vi "Client ATM machine.vi"() -> ()   [LabVIEW 2020]
uses:
  Sub VIs/Enum (Client).ctl
  <vilib>/regexp/Match Regular Expression.xnode
panel:
  out "Account no":string
  out "error out":errorcluster
  out "Data from server side":string caption="data out"
  out "First Name":string
  out "Balance":dbl
  out "Last Name":string
  in  "Client ATM Machine UI":enum32{"Page 1"}(tab)
  in  "User Input":string
  in  "Card Simulator":bool
  in  "Enter":bool
  out "ATM Message":string
  out "Left Menu":T1
  out "Right Menu":T2
  in  "Right Button":T3
  in  "Left Button":T4
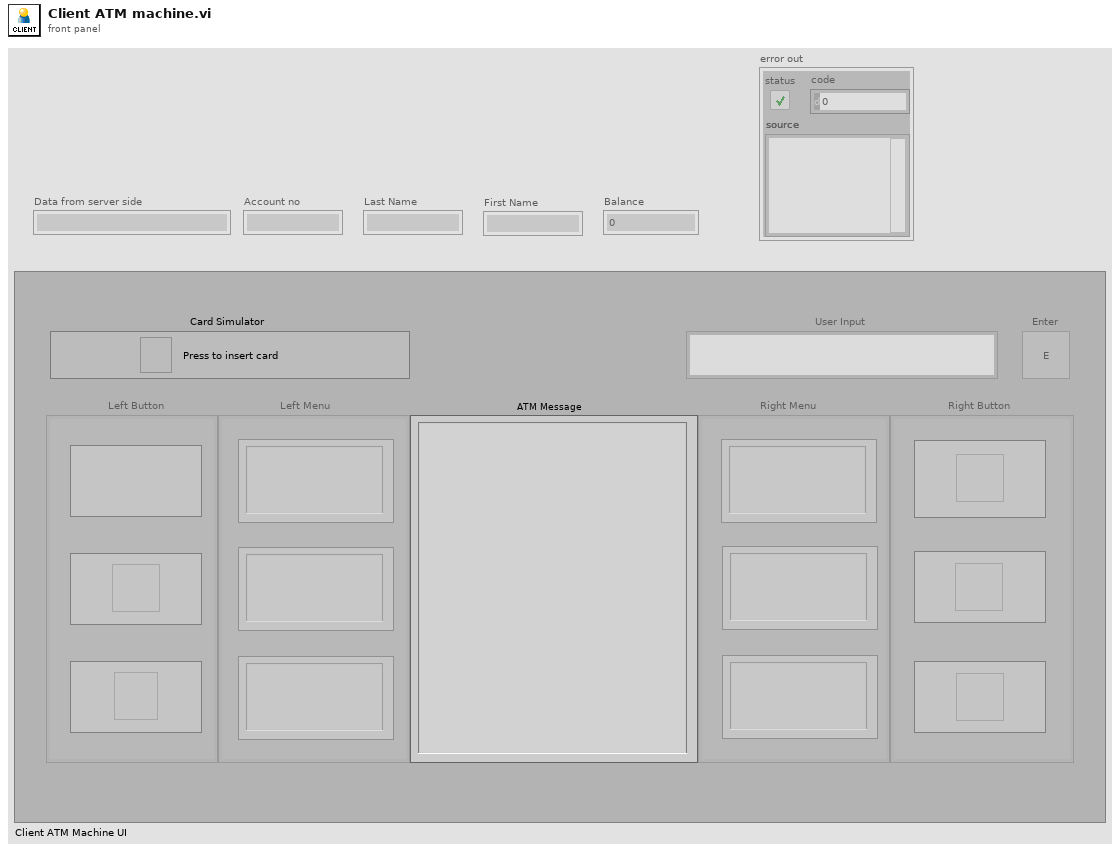
[diagram p1: front panel]
types:
  T1 = cluster{"Left Menu 3":string, "Left Menu 2":string, "Left Menu 4":string}
  T2 = cluster{"Right Menu 2":string, "Right Menu":string, "Right Menu 3":string}
  T3 = cluster{"Deposit":bool, "Withdraw":bool, "Fast Cash":bool}
  T4 = cluster{"None":bool, "Bank Inquires":bool, "Return Card and Terminate ":bool}
  T5 = typedef "Enum (Client).ctl" = enum16{"Start", "Idle", "Actions", "Empty Check", "Data Transmission", "Update File"}
  T6 = enum8{"Enabled", "Disabled", "Disabled and Grayed Out"}
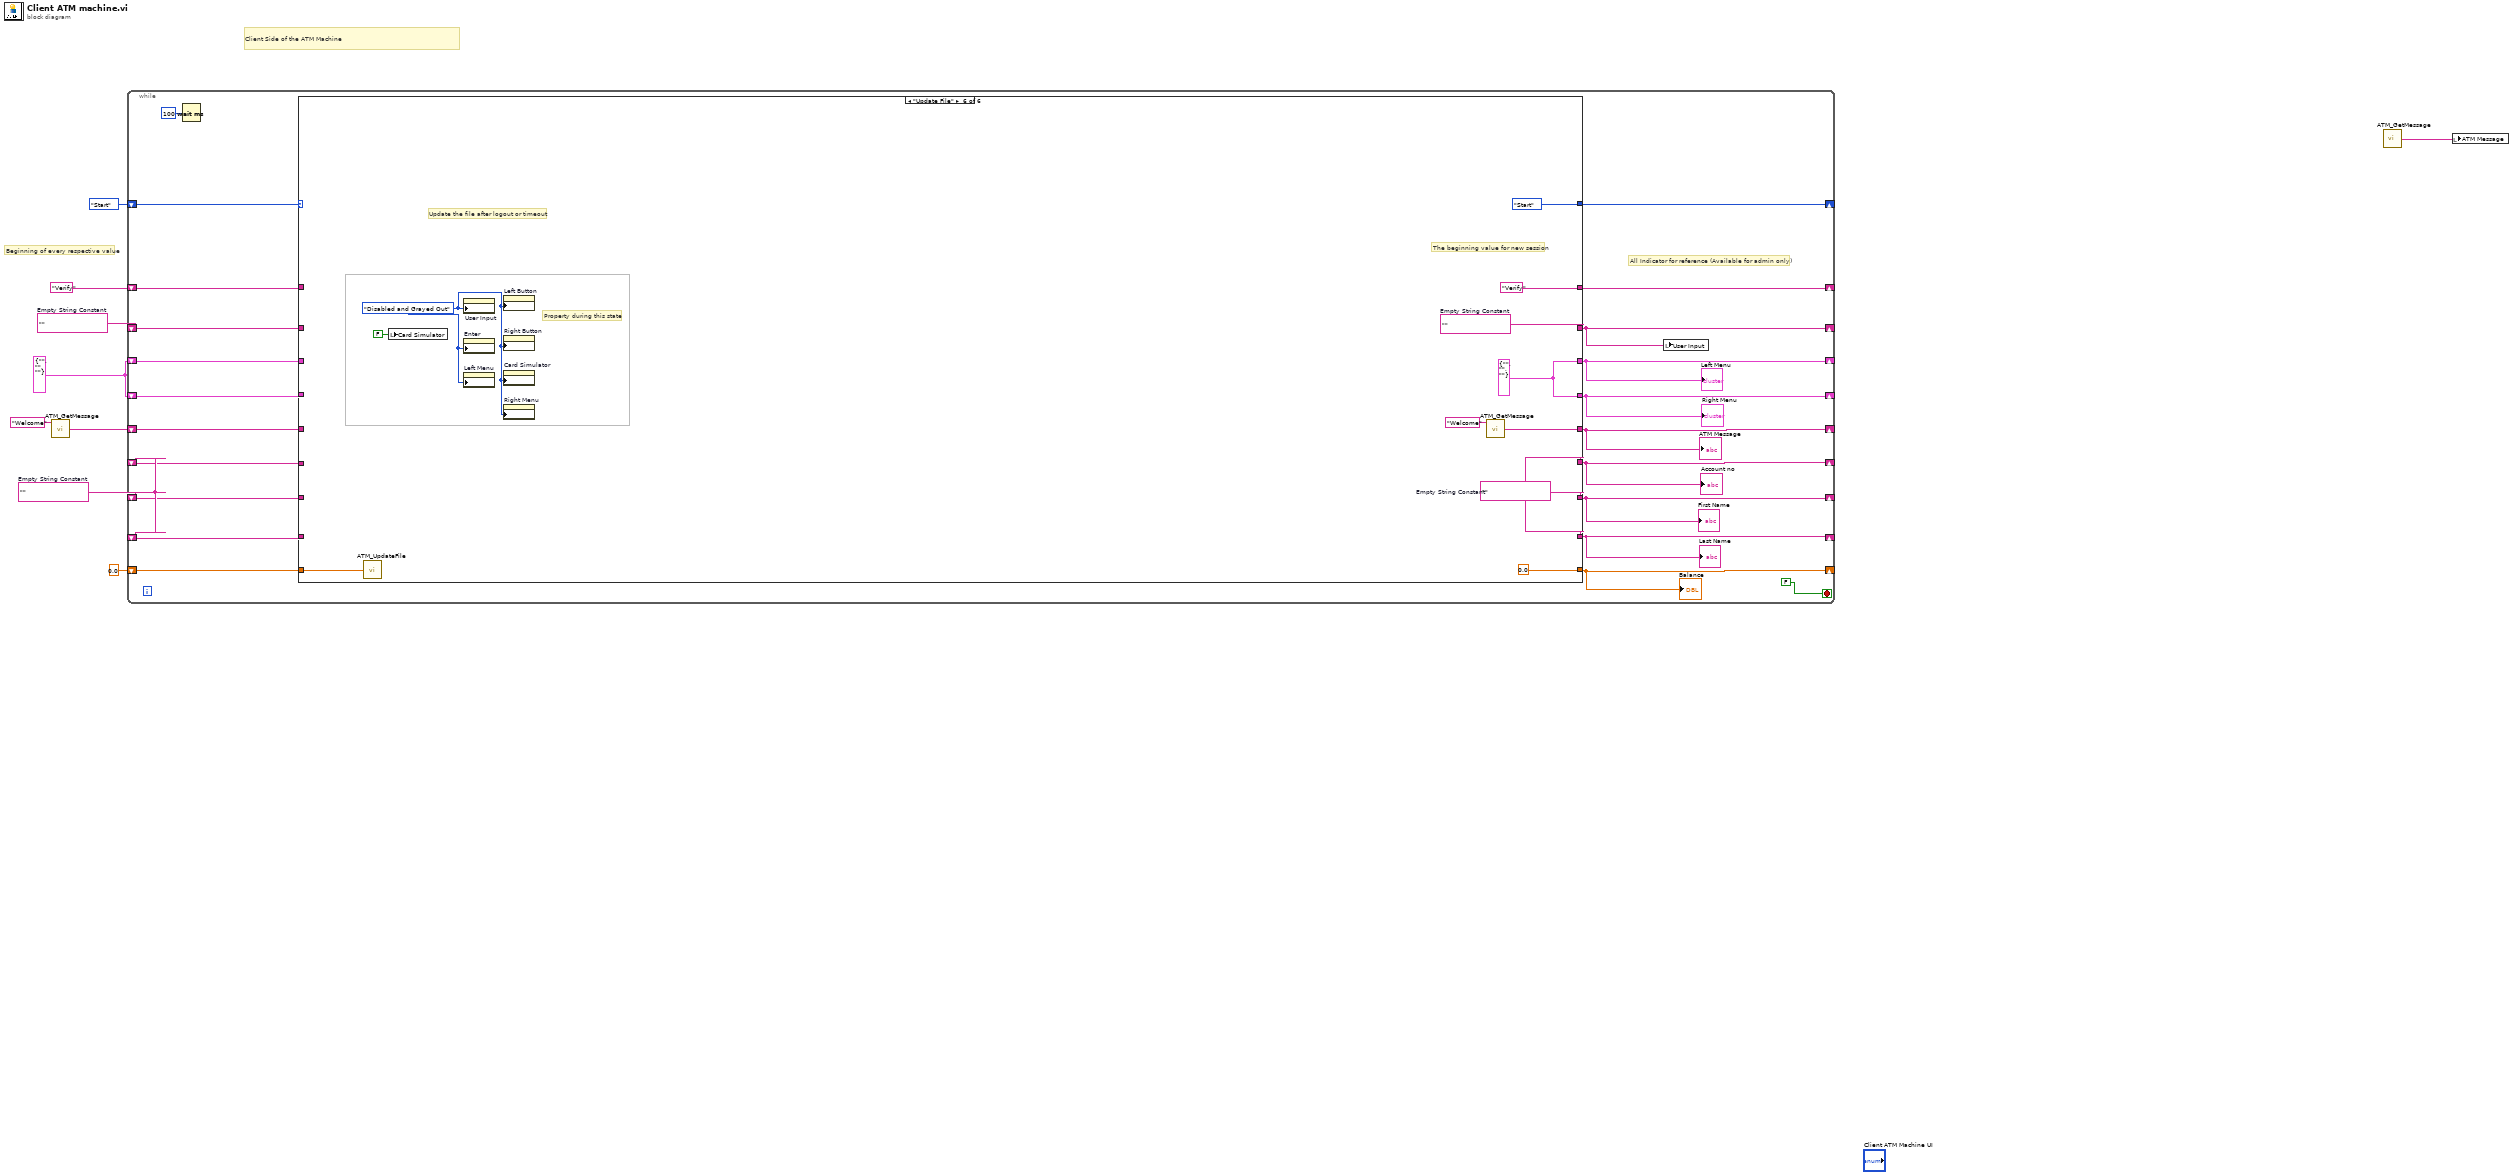
[diagram p0: block diagram]
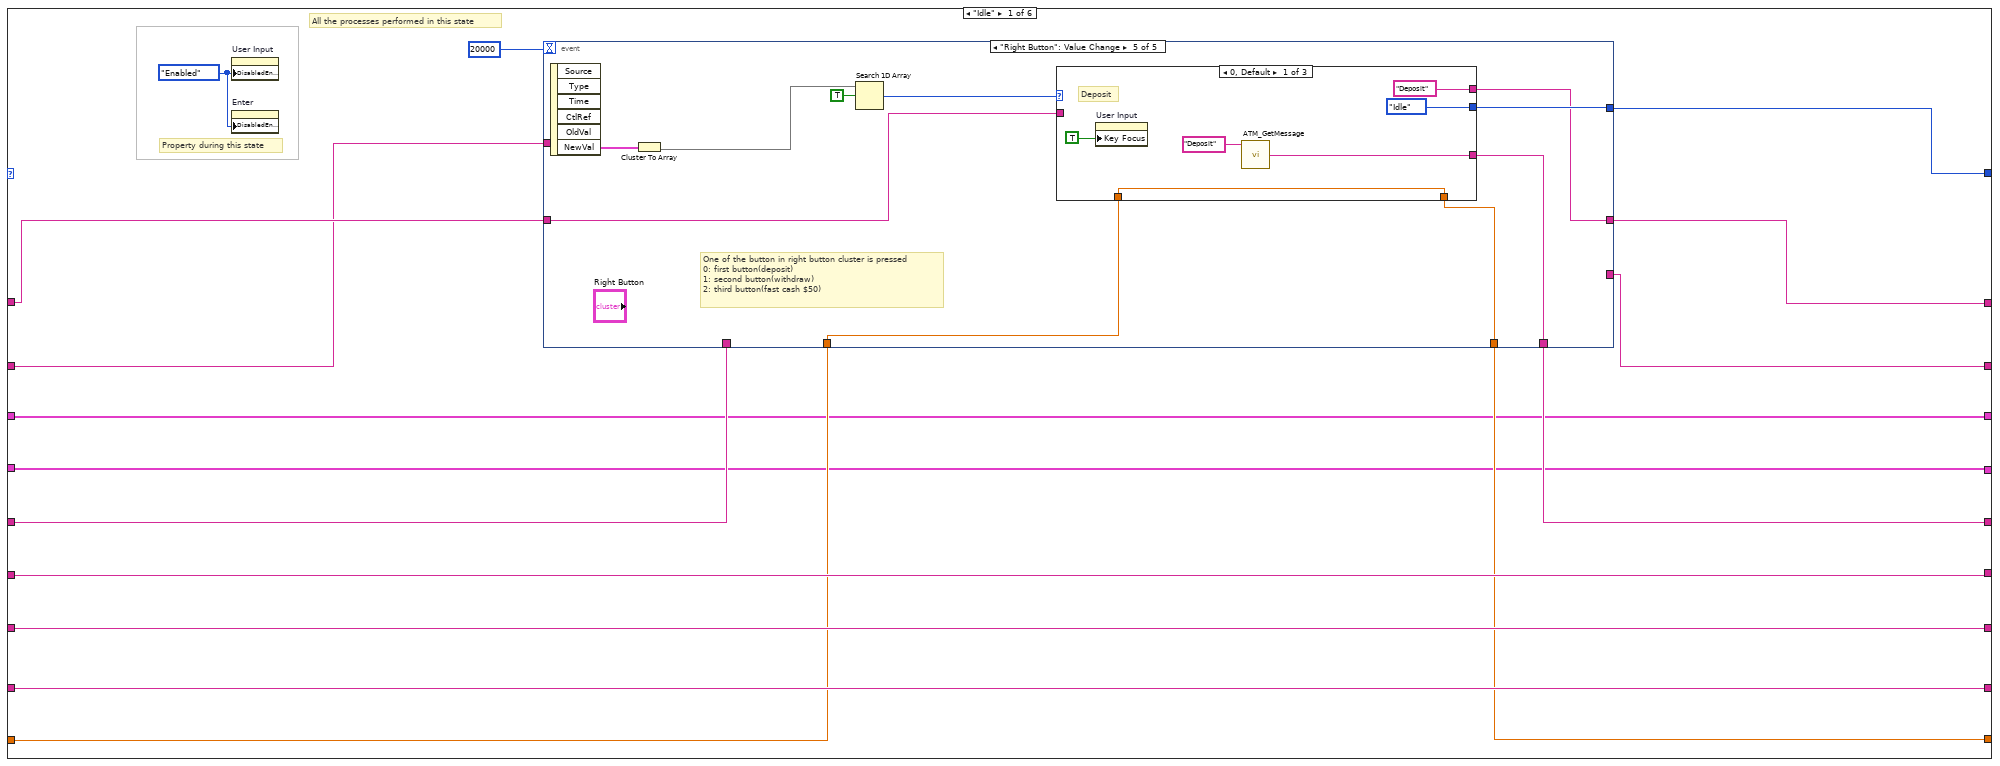
[diagram p2: hidden frame]
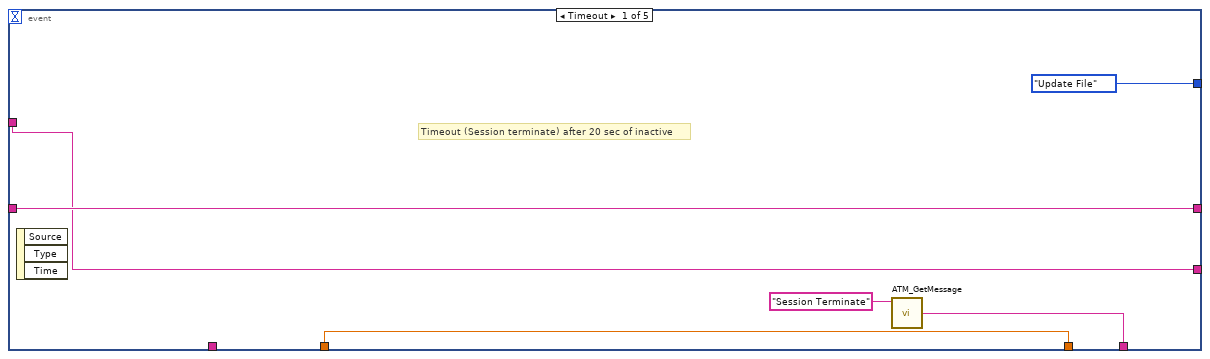
[diagram p3: hidden frame]
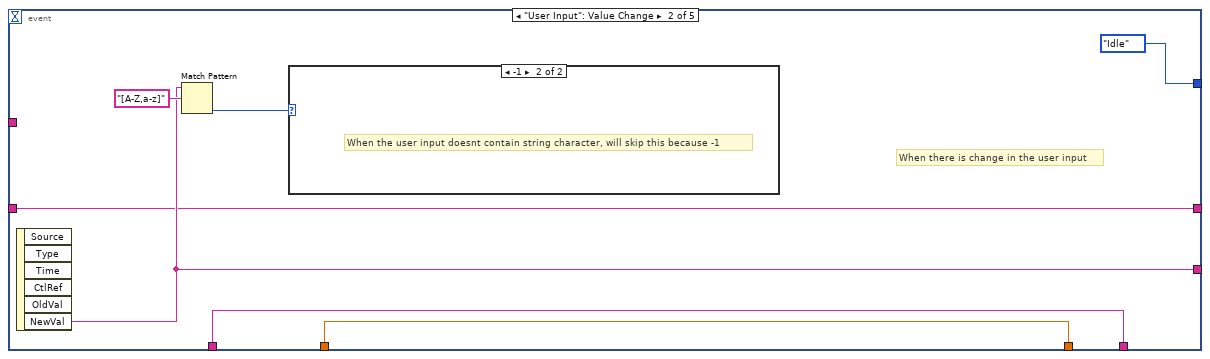
[diagram p4: hidden frame]
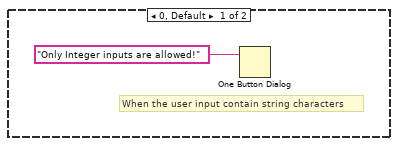
[diagram p5: hidden frame]
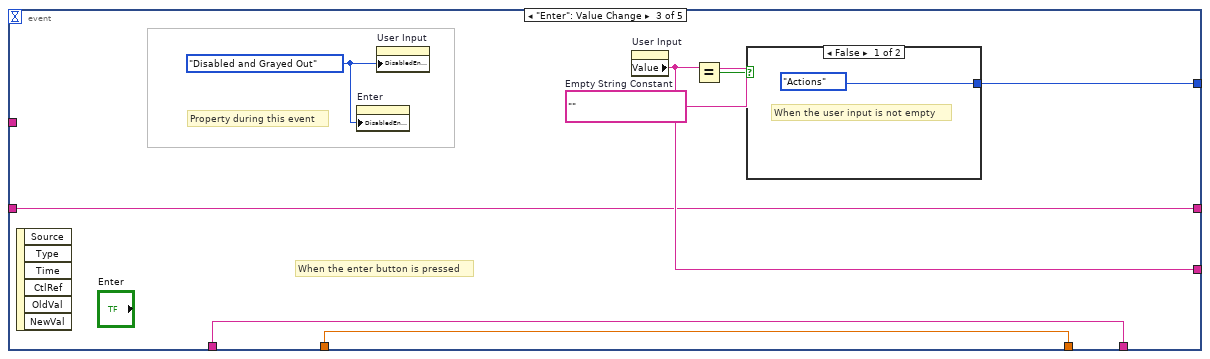
[diagram p6: hidden frame]
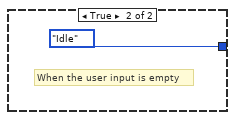
[diagram p7: hidden frame]
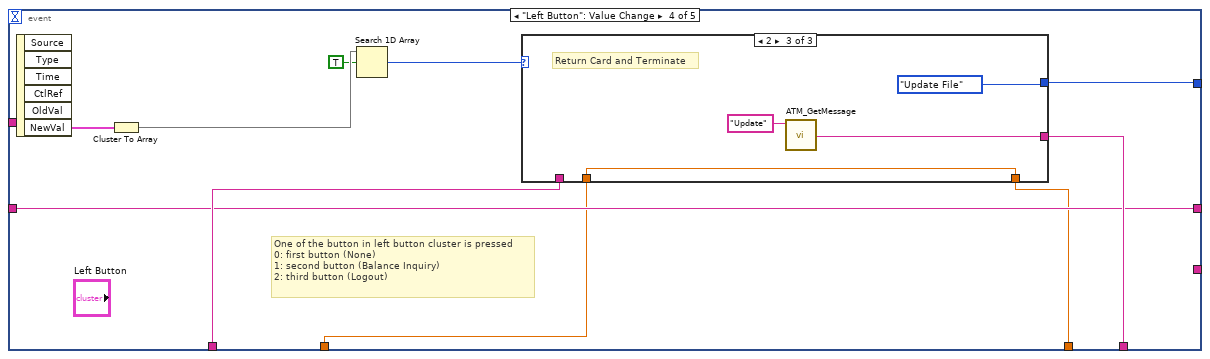
[diagram p8: hidden frame]
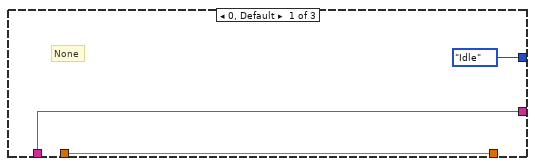
[diagram p9: hidden frame]
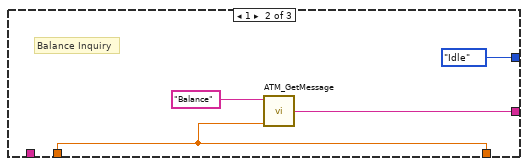
[diagram p10: hidden frame]
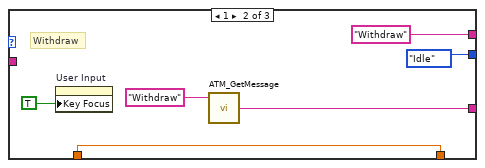
[diagram p11: hidden frame]
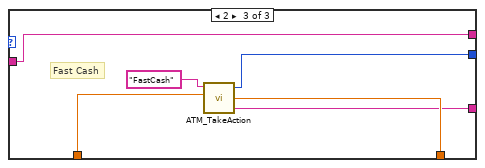
[diagram p12: hidden frame]
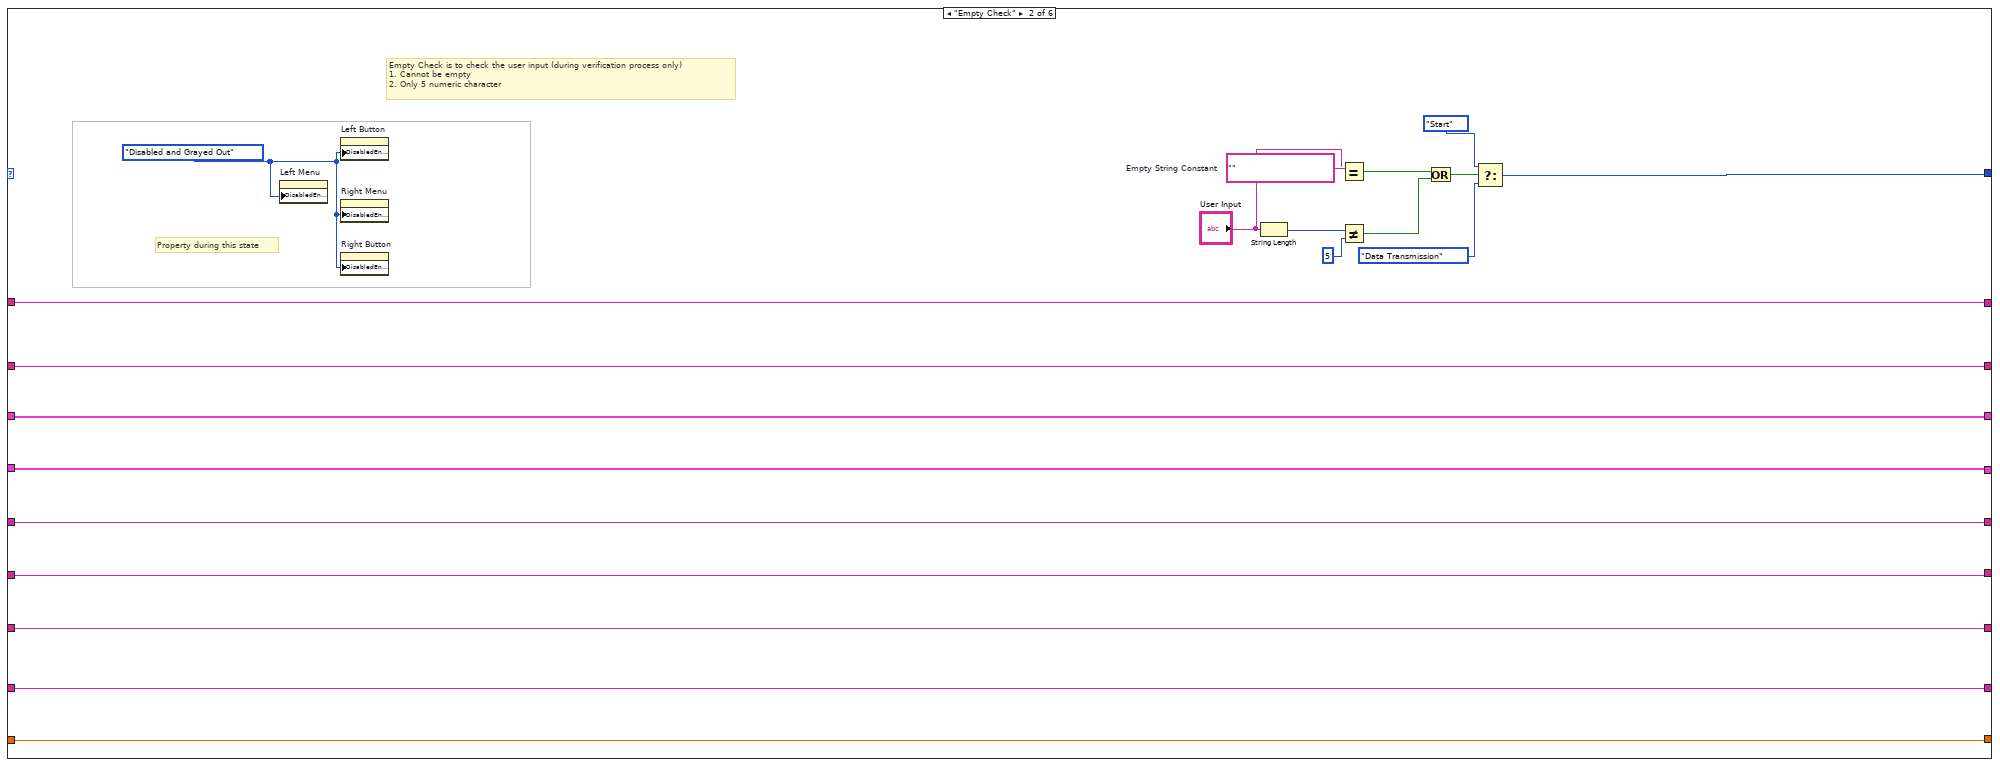
[diagram p13: hidden frame]
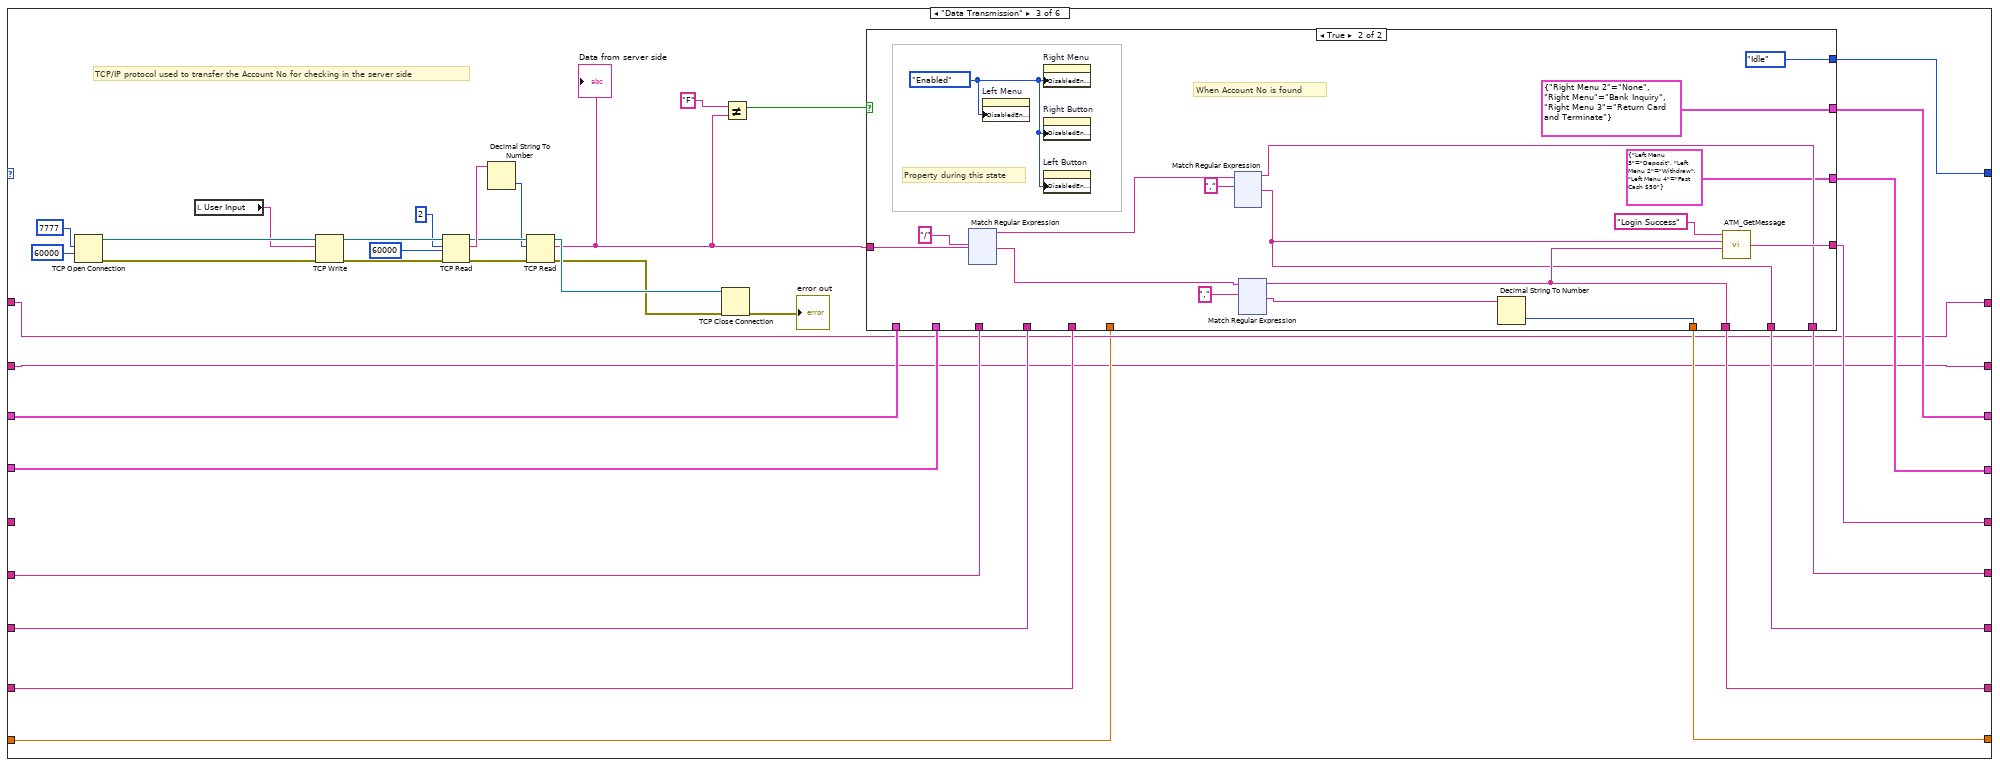
[diagram p14: hidden frame]
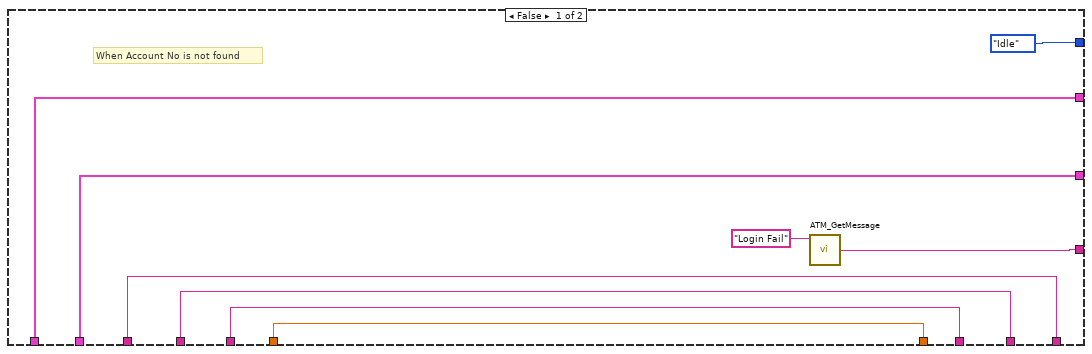
[diagram p15: hidden frame]
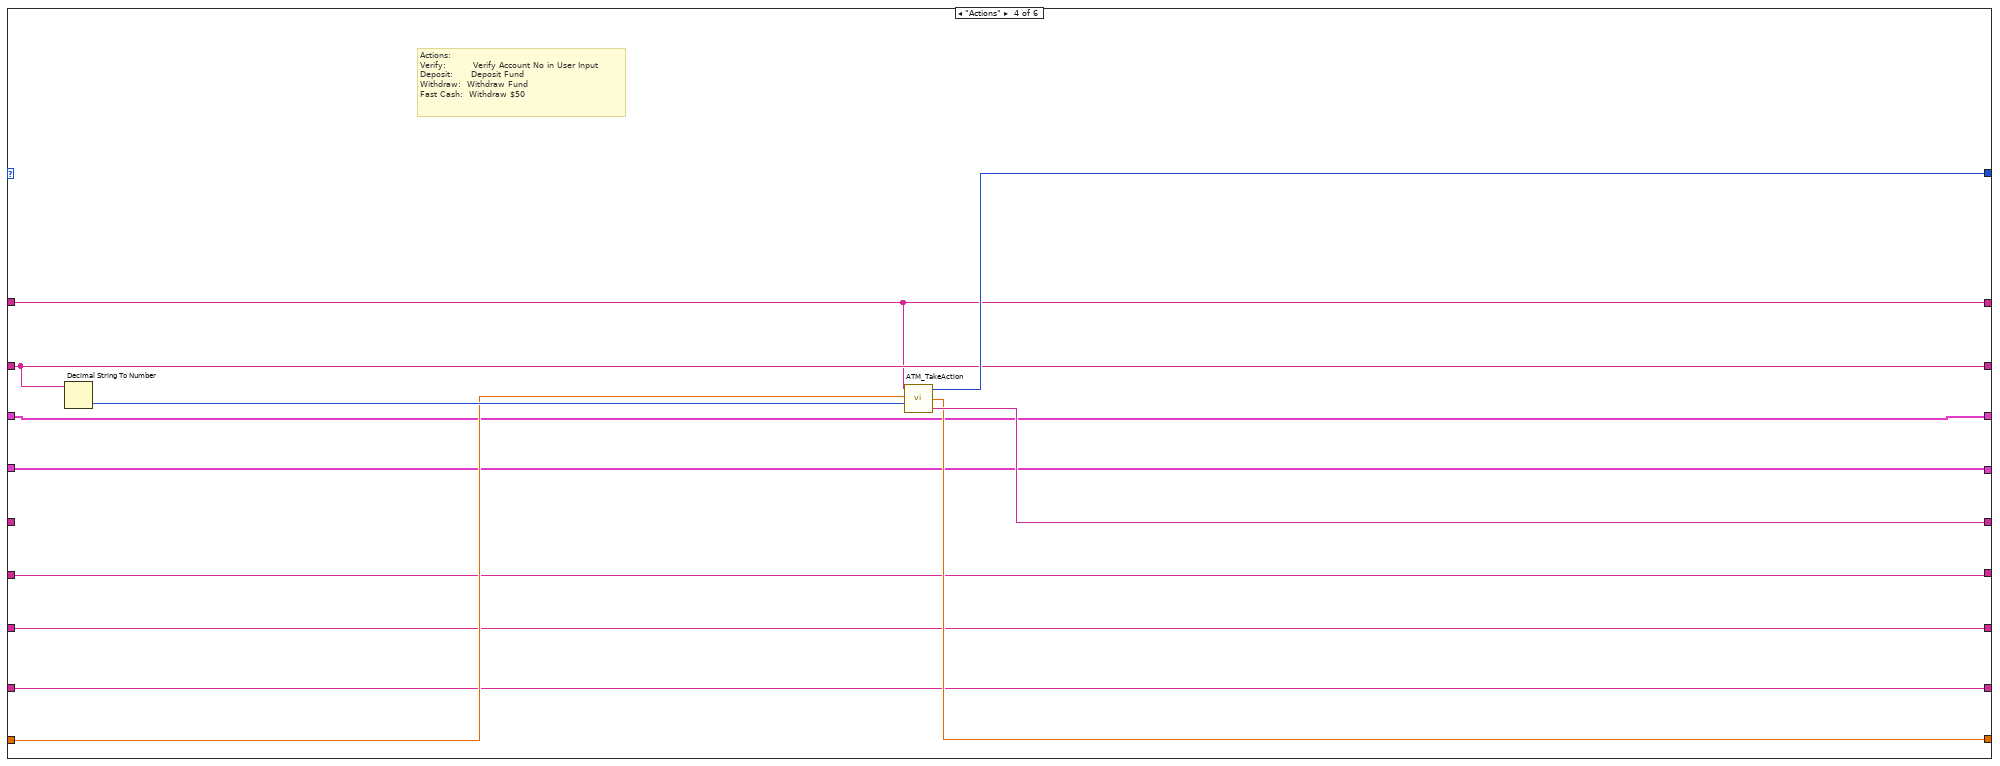
[diagram p16: hidden frame]
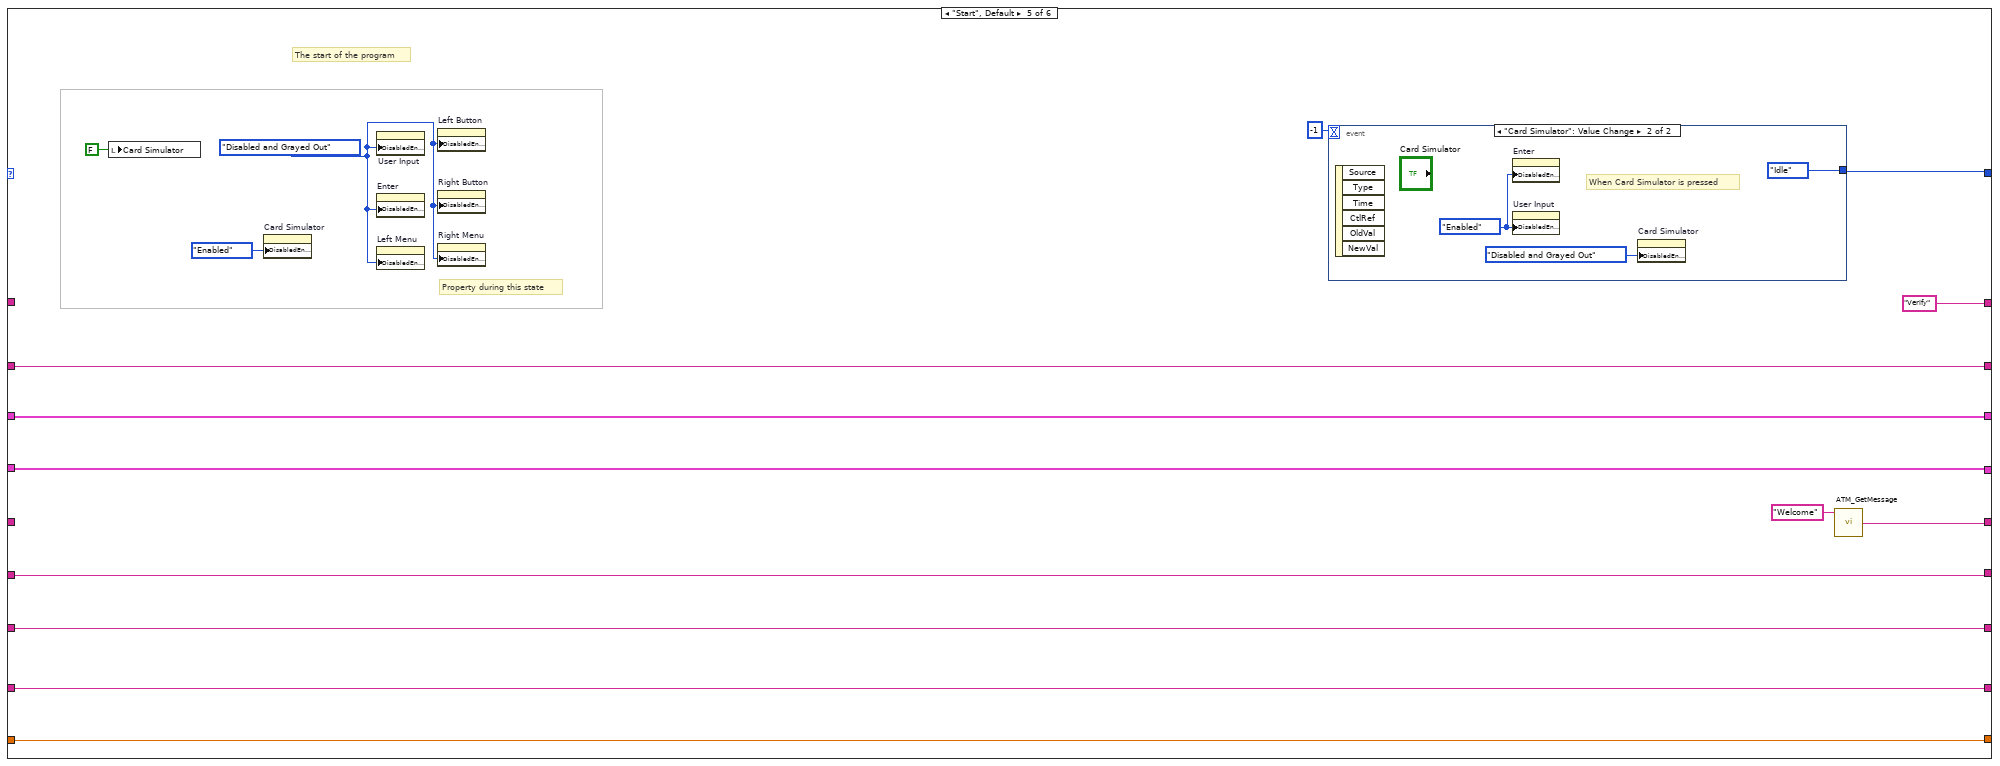
[diagram p17: hidden frame]
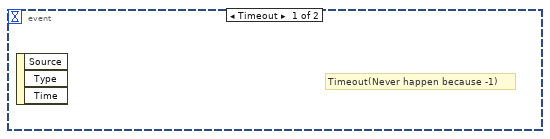
[diagram p18: hidden frame]
diagram:
  w1 = ""  # Empty String Constant
  w2 = ""  # Empty String Constant
  w6 = T2 {"Right Menu 2"="", "Right Menu"="", "Right Menu 3"=""} ("Right Menu")
  # "Client Side of the ATM Machine"
  # "Beginning of every respective value"
  n1 = call "ATM_GetMessage.vi"("Message Type"="Welcome") -> ("ATM Message"=w4:string)  [unwired: 4 in]
  n2 = while {
    shift-right: [w19] -> _
    shift-left: Enum_(Client)."Start" -> [w27]
    shift-right: [w28] -> _
    shift-left: "Verify" -> [w29]
    shift-right: [w16] -> _
    shift-left: w6 -> [w25]
    shift-right: [w18] -> _
    shift-left: w6 -> [w26]
    shift-right: [w20] -> _
    shift-left: 0.0 ("Balance") -> [w21]
    shift-right: [w13] -> _
    shift-left: w2 -> [w22]
    shift-right: [w15] -> _
    shift-left: w2 -> [w23]
    shift-right: [w17] -> _
    shift-left: w4 -> [w24]
    shift-right: [w11] -> _
    shift-left: w2 -> [w14]
    shift-right: [w10] -> _
    shift-left: w1 -> [w12]
    stop <- FALSE stop-if-true
    # "All Indicator for reference (Available for admin only)"
    n3 = Wait (ms)(milliseconds to wait=u32 100) -> ()  [unwired: 1 out]
    n4 = case shown="\"Update File\"" w27 {
      tunnel: [w47 w132 w141 w552 w560 Enum_(Client)."Start"] -> w19
      tunnel: w29 -> [w39 w131 w147 w544 _ _]
      tunnel: [w34 w131 w147 w544 "Verify" "Verify"] -> w28
      tunnel: [w44 w126 w159 w546 w564 w579] -> w13
      tunnel: [w46 w125 w158 w547 w563 w579] -> w15
      tunnel: [w43 w124 w157 w548 w567 w579] -> w11
      tunnel: [w42 w123 w156 w551 w568 0.0 ("Balance")] -> w20
      tunnel: [w36 w129 w155 w549 w566 w581] -> w18
      tunnel: [w37 w128 w154 w550 w565 w581] -> w16
      tunnel: w26 -> [w36 w129 w152 w549 w566 _]
      tunnel: w25 -> [w37 w128 w151 w550 w565 _]
      tunnel: w24 -> [w38 w127 _ _ _ _]
      tunnel: [w40 w127 w153 w553 w556 w574] -> w17
      tunnel: w23 -> [w46 w125 w149 w547 w563 _]
      tunnel: w22 -> [w44 w126 w150 w546 w564 _]
      tunnel: w21 -> [w41 w123 w146 w554 w568 w584]
      tunnel: w14 -> [w43 w124 w148 w548 w567 _]
      tunnel: w12 -> [w32 w122 w145 w545 w562 _]
      tunnel: [w35 w122 w145 w545 w562 w578] -> w10
      frame "Idle" {
        w33 = T6."Enabled" ("Disabled")
        # "Property during this state"
        # "All the processes performed in this state"
        n5 = property on="User Input" class="Str"("DisabledEnum"=w33) -> ()  [unwired: 2 in, 2 out]
        n6 = property on="Enter" class="Bool"("DisabledEnum"=w33) -> ()  [unwired: 2 in, 2 out]
        n7 = event shown="[4] \"Right Button\": Value Change" {
          selector: _ -> [_ _ _ _ _]
          dyn-events: _ -> [_ _ _ _ _]
          timeout: 20000 -> [_ _ _ _ _]
          tunnel: [Enum_(Client)."Update File" Enum_(Client)."Idle" w66 w77 w98] -> w47
          tunnel: w41 -> [w49 w58 w68 w73 w97]
          tunnel: [w49 w58 w68 w72 w96] -> w42
          tunnel: [w51 w57 w69 w76 w95] -> w40
          tunnel: w39 -> [w50 w55 w62 w74 w94]
          tunnel: w38 -> [_ w57 w69 w75 _]
          tunnel: [w48 w56 w64 _ _] -> w35
          tunnel: [w50 w55 w62 w74 w93] -> w34
          tunnel: w32 -> [w48 _ _ _ _]
          event Timeout {
            # "Timeout (Session terminate) after 20 sec of inactive"
            n8 = event-data() -> ()  [unwired: 1 in, 3 out]
            n9 = call "ATM_GetMessage.vi"("Message Type"="Session Terminate") -> ("ATM Message"=w51:string)  [unwired: 4 in]
          }
          event "User Input": Value Change {
            # "When there is change in the user input"
            n10 = event-data() -> ("NewVal"=w56:string)  [unwired: 1 in, 5 out]
            n11 = Match Pattern(string=w56, regular expression="[A-Z,a-z]") -> (offset past match=w60:i32)  [unwired: 1 in, 3 out]
            n12 = case shown="-1" w60 {
              frame 0, Default {
                # "When the user input contain string characters"
                n13 = One Button Dialog(message="Only Integer inputs are allowed!") -> ()  [unwired: 1 in, 1 out]
              }
              frame -1 {
                # "When the user input doesnt contain string character, will skip this because -1"
              }
            }
          }
          event "Enter": Value Change {
            w63 = T6."Disabled and Grayed Out" ("Disabled")
            w67 = ""  # Empty String Constant
            # "Property during this event"
            # "When the enter button is pressed"
            n14 = event-data() -> ()  [unwired: 1 in, 6 out]
            n15 = property on="Enter" class="Bool"("DisabledEnum"=w63) -> ()  [unwired: 2 in, 2 out]
            n16 = property on="User Input" class="Str"("DisabledEnum"=w63) -> ()  [unwired: 2 in, 2 out]
            n17 = property on="User Input" class="Str"() -> ("Value"=w64:string)  [unwired: 2 in, 2 out]
            n18 = Equal?(x=w64, y=w67) -> (x = y?=w65:bool)
            n19 = case shown="False" w65 {
              tunnel: [Enum_(Client)."Actions" Enum_(Client)."Idle"] -> w66
              frame False {
                # "When the user input is not empty"
              }
              frame True {
                # "When the user input is empty"
              }
            }
          }
          event "Left Button": Value Change {
            # "One of the button in left button cluster is pressed\n0: first button (None)\n1: second button (Balance Inquiry)\n2: third button (Logout)"
            n20 = event-data() -> ("NewVal"=w78:T4)  [unwired: 1 in, 5 out]
            n21 = Cluster To Array(cluster=w78) -> (array=w81:bool[])
            n22 = Search 1D Array(1D array=w81, element=TRUE) -> (index of element=w79:i32)  [unwired: 1 in]
            n23 = case shown="2" w79 {
              tunnel: [Enum_(Client)."Idle" Enum_(Client)."Idle" Enum_(Client)."Update File"] -> w77
              tunnel: [w82 w85 w89] -> w72
              tunnel: [w83 w86 w90] -> w76
              tunnel: w75 -> [w83 _ _]
              tunnel: w73 -> [w82 w85 w89]
              frame 0, Default {
                # "None"
              }
              frame 1 {
                # "Balance Inquiry"
                n24 = call "ATM_GetMessage.vi"("Message Type"="Balance", "Balance"=w85) -> ("ATM Message"=w86:string)  [unwired: 3 in]
              }
              frame 2 {
                # "Return Card and Terminate"
                n25 = call "ATM_GetMessage.vi"("Message Type"="Update") -> ("ATM Message"=w90:string)  [unwired: 4 in]
              }
            }
          }
          event "Right Button": Value Change {
            # "One of the button in right button cluster is pressed\n0: first button(deposit)\n1: second button(withdraw)\n2: third button(fast cash $50)"
            n26 = event-data() -> ("NewVal"=w99:T3)  [unwired: 1 in, 5 out]
            n27 = Cluster To Array(cluster=w99) -> (array=w102:bool[])
            n28 = Search 1D Array(1D array=w102, element=TRUE) -> (index of element=w101:i32)  [unwired: 1 in]
            n29 = case shown="0, Default" w101 {
              tunnel: ["Deposit" "Withdraw" w115] -> w93
              tunnel: [Enum_(Client)."Idle" Enum_(Client)."Idle" w119] -> w98
              tunnel: w97 -> [w106 w111 w118]
              tunnel: [w106 w111 w117] -> w96
              tunnel: [w105 w110 w116] -> w95
              tunnel: w94 -> [_ _ w115]
              frame 0, Default {
                # "Deposit"
                n30 = property on="User Input" class="Str"("Key Focus"=TRUE) -> ()  [unwired: 2 in, 2 out]
                n31 = call "ATM_GetMessage.vi"("Message Type"="Deposit") -> ("ATM Message"=w105:string)  [unwired: 4 in]
              }
              frame 1 {
                # "Withdraw"
                n32 = property on="User Input" class="Str"("Key Focus"=TRUE) -> ()  [unwired: 2 in, 2 out]
                n33 = call "ATM_GetMessage.vi"("Message Type"="Withdraw") -> ("ATM Message"=w110:string)  [unwired: 4 in]
              }
              frame 2 {
                # "Fast Cash"
                n34 = call "ATM_TakeAction.vi"("Balance"=w118, "Action Type"="FastCash") -> ("ATM Message"=w116:string, "New Balance"=w117:dbl, "Enum"=w119:T5)  [unwired: 2 in]
              }
            }
          }
        }
      }
      frame "Empty Check" {
        w121 = T6."Disabled and Grayed Out" ("Disabled")
        w140 = ""  # Empty String Constant
        # "Property during this state"
        # "Empty Check is to check the user input (during verification process only) \n1. Cannot be empty\n2. Only 5 numeric character"
        n35 = property on="Left Menu" class="Clust (strict)"("DisabledEnum"=w121) -> ()  [unwired: 2 in, 2 out]
        n36 = property on="Left Button" class="Clust"("DisabledEnum"=w121) -> ()  [unwired: 2 in, 2 out]
        n37 = property on="Right Menu" class="Clust (strict)"("DisabledEnum"=w121) -> ()  [unwired: 2 in, 2 out]
        n38 = property on="Right Button" class="Clust"("DisabledEnum"=w121) -> ()  [unwired: 2 in, 2 out]
        n39 = String Length(string="User Input") -> (length=w139:i32)
        n40 = Equal?(x="User Input", y=w140) -> (x = y?=w137:bool)
        n41 = Not Equal?(x=w139, y=5) -> (x != y?=w136:bool)
        n42 = Or(x=w137, y=w136) -> (x .or. y?=w135:bool)
        n43 = Select(t=Enum_(Client)."Start", s=w135, f=Enum_(Client)."Data Transmission") -> (s? t:f=w132:T5)
      }
      frame "Data Transmission" {
        # "TCP/IP protocol used to transfer the Account No for checking in the server side"
        n44 = TCP Open Connection(remote port or service name=u16 7777, timeout ms (60000)=60000) -> (connection ID=w175:refnum<k5>, error out=w169:errorcluster)  [unwired: 3 in]
        n45 = local read "User Input"() -> (w144:string)
        n46 = TCP Write(connection ID=w175, data in=w144, error in (no error)=w169) -> (connection ID out=w172:refnum<k5>, error out=w168:errorcluster)  [unwired: 1 in, 1 out]
        n47 = TCP Read(connection ID=w172, bytes to read=2, error in (no error)=w168, 9:60000 ("timeout ms (25000)")) -> (connection ID out=w165:refnum<k5>, data out=w170:string, error out=w163:errorcluster)  [unwired: 1 in]
        n48 = Decimal String To Number(string=w170) -> (number=w164:i32)  [unwired: 2 in, 1 out]
        n49 = TCP Read(connection ID=w165, bytes to read=w164, error in (no error)=w163) -> (connection ID out=w166:refnum<k5>, data out=w143:string, error out=w162:errorcluster)  [unwired: 2 in]
        "Data from server side" <- w143
        n50 = TCP Close Connection(connection ID=w166, error in (no error)=w162) -> (error out=→"error out":errorcluster)  [unwired: 1 in, 1 out]
        n51 = Not Equal?(x="F" ("y"), y=w143) -> (x != y?=w160:bool)
        n52 = case shown="True" w160 {
          tunnel: [Enum_(Client)."Idle" Enum_(Client)."Idle"] -> w141
          tunnel: w143 -> [_ w199]
          tunnel: [w183 w192] -> w153
          tunnel: [w179 w191] -> w159
          tunnel: [w178 w185] -> w158
          tunnel: [w177 w186] -> w157
          tunnel: [w176 w190] -> w156
          tunnel: [w181 T2 {"Right Menu 2"="None", "Right Menu"="Bank Inquiry", "Right Menu 3"="Return Card and Terminate"} ("Right Menu")] -> w155
          tunnel: [w180 T1 {"Left Menu 3"="Deposit", "Left Menu 2"="Withdraw", "Left Menu 4"="Fast Cash $50"} ("Left Menu")] -> w154
          tunnel: w152 -> [w181 _]
          tunnel: w151 -> [w180 _]
          tunnel: w150 -> [w179 _]
          tunnel: w149 -> [w178 _]
          tunnel: w148 -> [w177 _]
          tunnel: w146 -> [w176 _]
          frame False {
            # "When Account No is not found"
            n53 = call "ATM_GetMessage.vi"("Message Type"="Login Fail") -> ("ATM Message"=w183:string)  [unwired: 4 in]
          }
          frame True {
            w187 = T6."Enabled" ("Disabled")
            # "Property during this state"
            # "When Account No is found"
            n54 = xnode "Match Regular Expression"("input string"=w199, "regular expression"="/") -> ("before match"=w197:string, "after match"=w195:string)  [unwired: 4 in, 3 out]
            n55 = property on="Left Menu" class="Clust (strict)"("DisabledEnum"=w187) -> ()  [unwired: 2 in, 2 out]
            n56 = property on="Right Menu" class="Clust (strict)"("DisabledEnum"=w187) -> ()  [unwired: 2 in, 2 out]
            n57 = property on="Right Button" class="Clust"("DisabledEnum"=w187) -> ()  [unwired: 2 in, 2 out]
            n58 = property on="Left Button" class="Clust"("DisabledEnum"=w187) -> ()  [unwired: 2 in, 2 out]
            n59 = xnode "Match Regular Expression"("input string"=w197, "regular expression"=",") -> ("before match"=w191:string, "after match"=w185:string)  [unwired: 4 in, 3 out]
            n60 = xnode "Match Regular Expression"("input string"=w195, "regular expression"=",") -> ("before match"=w186:string, "after match"=w193:string)  [unwired: 4 in, 3 out]
            n61 = Decimal String To Number(string=w193) -> (number=w190:i32)  [unwired: 2 in, 1 out]
            n62 = call "ATM_GetMessage.vi"("Message Type"="Login Success", "First Name"=w185, "Last Name"=w186) -> ("ATM Message"=w192:string)  [unwired: 2 in]
          }
        }
      }
      frame "Actions" {
        # "Actions:\nVerify:         Verify Account No in User Input\nDeposit:      Deposit Fund\nWithdraw:  Withdraw Fund\nFast Cash:  Withdraw $50"
        n63 = Decimal String To Number(string=w545) -> (number=w555:i32)  [unwired: 2 in, 1 out]
        n64 = call "ATM_TakeAction.vi"("User Input"=w555, "Balance"=w554, "Action Type"=w544) -> ("ATM Message"=w553:string, "New Balance"=w551:dbl, "Enum"=w552:T5)  [unwired: 1 in]
      }
      frame "Start", Default {
        w570 = T6."Disabled and Grayed Out" ("Disabled")
        # "Property during this state"
        # "The start of the program"
        n65 = local write "Card Simulator"(FALSE ("Card Simulator")) -> ()
        n66 = property on="Card Simulator" class="Bool (strict)"("DisabledEnum"=T6."Enabled" ("Disabled")) -> ()  [unwired: 2 in, 2 out]
        n67 = property on="User Input" class="Str"("DisabledEnum"=w570) -> ()  [unwired: 2 in, 2 out]
        n68 = property on="Enter" class="Bool"("DisabledEnum"=w570) -> ()  [unwired: 2 in, 2 out]
        n69 = property on="Left Menu" class="Clust (strict)"("DisabledEnum"=w570) -> ()  [unwired: 2 in, 2 out]
        n70 = property on="Left Button" class="Clust"("DisabledEnum"=w570) -> ()  [unwired: 2 in, 2 out]
        n71 = property on="Right Button" class="Clust"("DisabledEnum"=w570) -> ()  [unwired: 2 in, 2 out]
        n72 = property on="Right Menu" class="Clust (strict)"("DisabledEnum"=w570) -> ()  [unwired: 2 in, 2 out]
        n73 = event shown="[1] \"Card Simulator\": Value Change" {
          selector: _ -> [_ _]
          dyn-events: _ -> [_ _]
          timeout: -1 -> [_ _]
          tunnel: [_ Enum_(Client)."Idle"] -> w560
          event Timeout {
            # "Timeout(Never happen because -1)"
            n74 = event-data() -> ()  [unwired: 1 in, 3 out]
          }
          event "Card Simulator": Value Change {
            w573 = T6."Enabled" ("Disabled")
            # "When Card Simulator is pressed"
            n75 = event-data() -> ()  [unwired: 1 in, 6 out]
            n76 = property on="Enter" class="Bool"("DisabledEnum"=w573) -> ()  [unwired: 2 in, 2 out]
            n77 = property on="User Input" class="Str"("DisabledEnum"=w573) -> ()  [unwired: 2 in, 2 out]
            n78 = property on="Card Simulator" class="Bool (strict)"("DisabledEnum"=T6."Disabled and Grayed Out" ("Disabled")) -> ()  [unwired: 2 in, 2 out]
          }
        }
        n79 = call "ATM_GetMessage.vi"("Message Type"="Welcome") -> ("ATM Message"=w556:string)  [unwired: 4 in]
      }
      frame "Update File" {
        w576 = T6."Disabled and Grayed Out" ("Disabled")
        w578 = ""  # Empty String Constant
        w579 = ""  # Empty String Constant
        w581 = T2 {"Right Menu 2"="", "Right Menu"="", "Right Menu 3"=""} ("Right Menu")
        # "Property during this state"
        # "The beginning value for new session"
        # "Update the file after logout or timeout"
        n80 = call "ATM_UpdateFile.vi"("Balance"=w584) -> ()
        n81 = local write "Card Simulator"(FALSE ("Card Simulator")) -> ()
        n82 = property on="User Input" class="Str"("DisabledEnum"=w576) -> ()  [unwired: 2 in, 2 out]
        n83 = property on="Enter" class="Bool"("DisabledEnum"=w576) -> ()  [unwired: 2 in, 2 out]
        n84 = property on="Left Menu" class="Clust (strict)"("DisabledEnum"=w576) -> ()  [unwired: 2 in, 2 out]
        n85 = property on="Left Button" class="Clust"("DisabledEnum"=w576) -> ()  [unwired: 2 in, 2 out]
        n86 = property on="Right Button" class="Clust"("DisabledEnum"=w576) -> ()  [unwired: 2 in, 2 out]
        n87 = property on="Card Simulator" class="Bool (strict)"("DisabledEnum"=w576) -> ()  [unwired: 2 in, 2 out]
        n88 = property on="Right Menu" class="Clust (strict)"("DisabledEnum"=w576) -> ()  [unwired: 2 in, 2 out]
        n89 = call "ATM_GetMessage.vi"("Message Type"="Welcome") -> ("ATM Message"=w574:string)  [unwired: 4 in]
      }
    }
    "ATM Message" <- w17
    "Account no" <- w13
    "First Name" <- w15
    "Last Name" <- w11
    "Balance" <- w20
    "Left Menu" <- w18
    "Right Menu" <- w16
    n90 = local write "User Input"(w10) -> ()
  }
  n91 = call "ATM_GetMessage.vi"() -> ("ATM Message"=w9:string)  [unwired: 5 in]
  n92 = local write "ATM Message"(w9) -> ()
